vi "get serial number.vi"(8 "error in (no error)":errorcluster, 10 "SerialNumber":u32, 11 "id":i32) -> (0 "error out":errorcluster, 2 "SerialNumber out":u32, 3 "function return":i32)   [LabVIEW 2020, in "libximc.lvlib"]
doc: "result_t XIMC_API get_serial_number (device_t id, unsigned int* SerialNumber);"
uses:
  libximc.lvlib
  libximc.dll
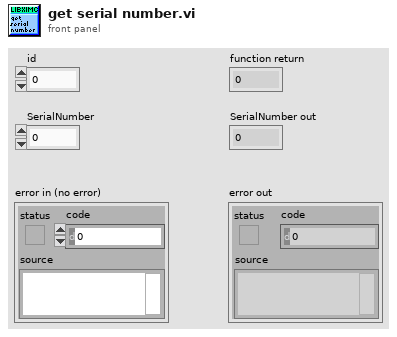
[diagram p1: front panel]
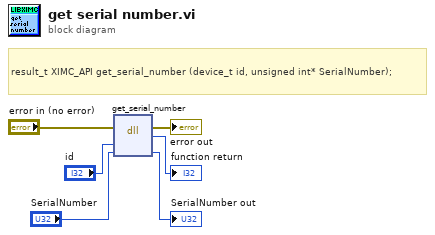
[diagram p0: block diagram]
diagram:
  # "result_t XIMC_API get_serial_number (device_t id, unsigned int* SerialNumber);"
  n1 = dll-call lib="E:/Norway Project/All Hardware/New Microscope/LabVIEW/Stage/libximc.*" fn="get_serial_number"(error in="error in (no error)", "id"="id", "SerialNumber"="SerialNumber") -> (error out=→"error out":errorcluster, →"function return":i32, "SerialNumber"=→"SerialNumber out":u32)  [unwired: 3 in, 1 out]
